vi "Experiment.vi"() -> ()   [LabVIEW 2016]
uses:
  controls/Enum.ctl
  <vilib>/rvi/interface/nirviOpenFPGA/nirviOpenFPGA.xnode
  controls/FPGAVIreferenceTypeDef.ctl
  Course Project/support/Message Queue/Message Queue.lvlib
  <vilib>/rvi/interface/nirviReadWriteControl/nirviReadWriteControl.xnode
  controls/FPGAVIreferenceTypeDefScanEngine.ctl
  <vilib>/FPGAPlugInAG/USB-7856R OEM/niLvFpga_Open_USB-7856R OEM.vi
  FPGA Bitfiles/qnmController797_usbRIO_controllerFPGAmu.lvbitx
  FPGA Bitfiles/lbniAFMControlle_scanControl2_controllerFPGAPX_D62jLejMcas.lvbitx
  controllerFPGA_multiTarget.vi
  <vilib>/FPGAPlugInAG/PXI-7842R/niLvFpga_Open_PXI-7842R.vi
  NiFpgaLv.dll
  <vilib>/rvi/errors/niLvFpgaAdjustHostInterfaceError.vi
  controls/Monitor.ctl
panel:
  in  "Head":i32(listbox)
  in  "Actions":T1
  out "Image":T2
  out "Profileh":dbl[][](graph)
  in  "Scan Engine":i32[](listbox)
  in  "FPGA":i32[](listbox)
  in  "Experiment":i32(listbox)
  in  "Microscope":i32(listbox)
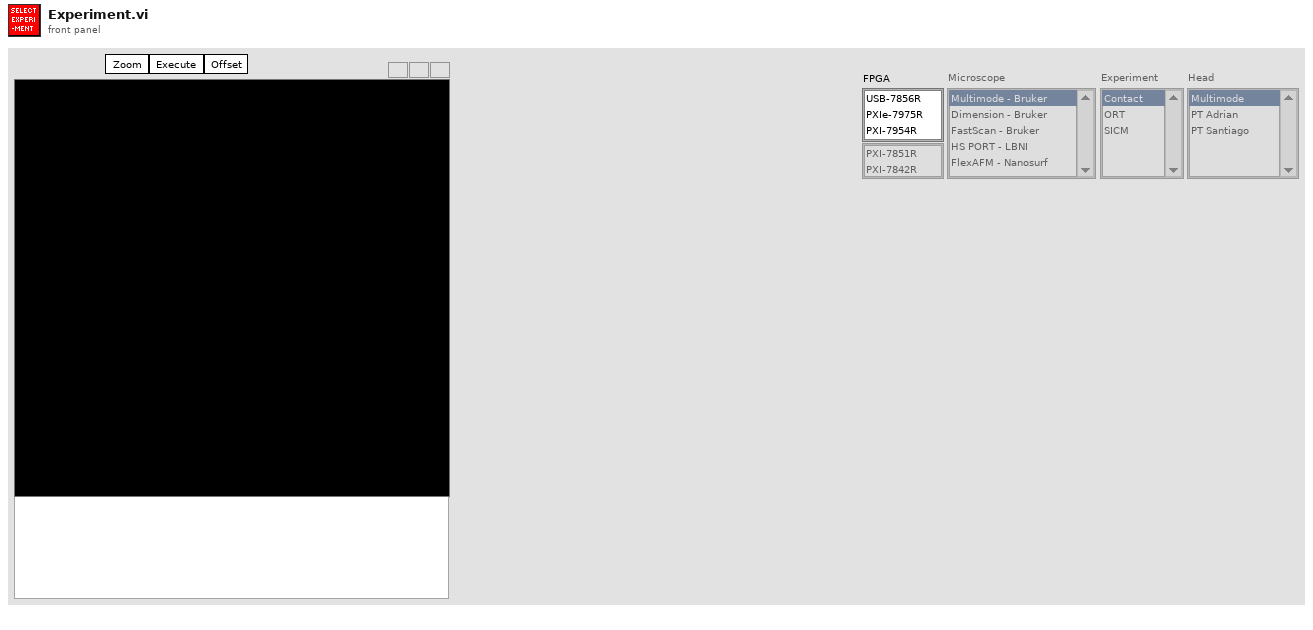
[diagram p1: front panel]
types:
  T1 = cluster{"Zoom":bool, "Execute":bool, "Offset":bool}
  T2 = typedef "Monitor.ctl" = dbl[][]
  T3 = typedef "Message Queue.lvlib/All Message Queues.ctl" = cluster{"IU":refnum<queue>}
  T4 = enum8{"Enabled", "Disabled", "Disabled and Grayed Out"}
  T5 = typedef "Enum.ctl" = enum16{"Init", "Read", "Write"}
  T6 = typedef "FPGAVIreferenceTypeDef.ctl" = refnum<k20>
  T7 = typedef "FPGAVIreferenceTypeDefScanEngine.ctl" = refnum<k20>
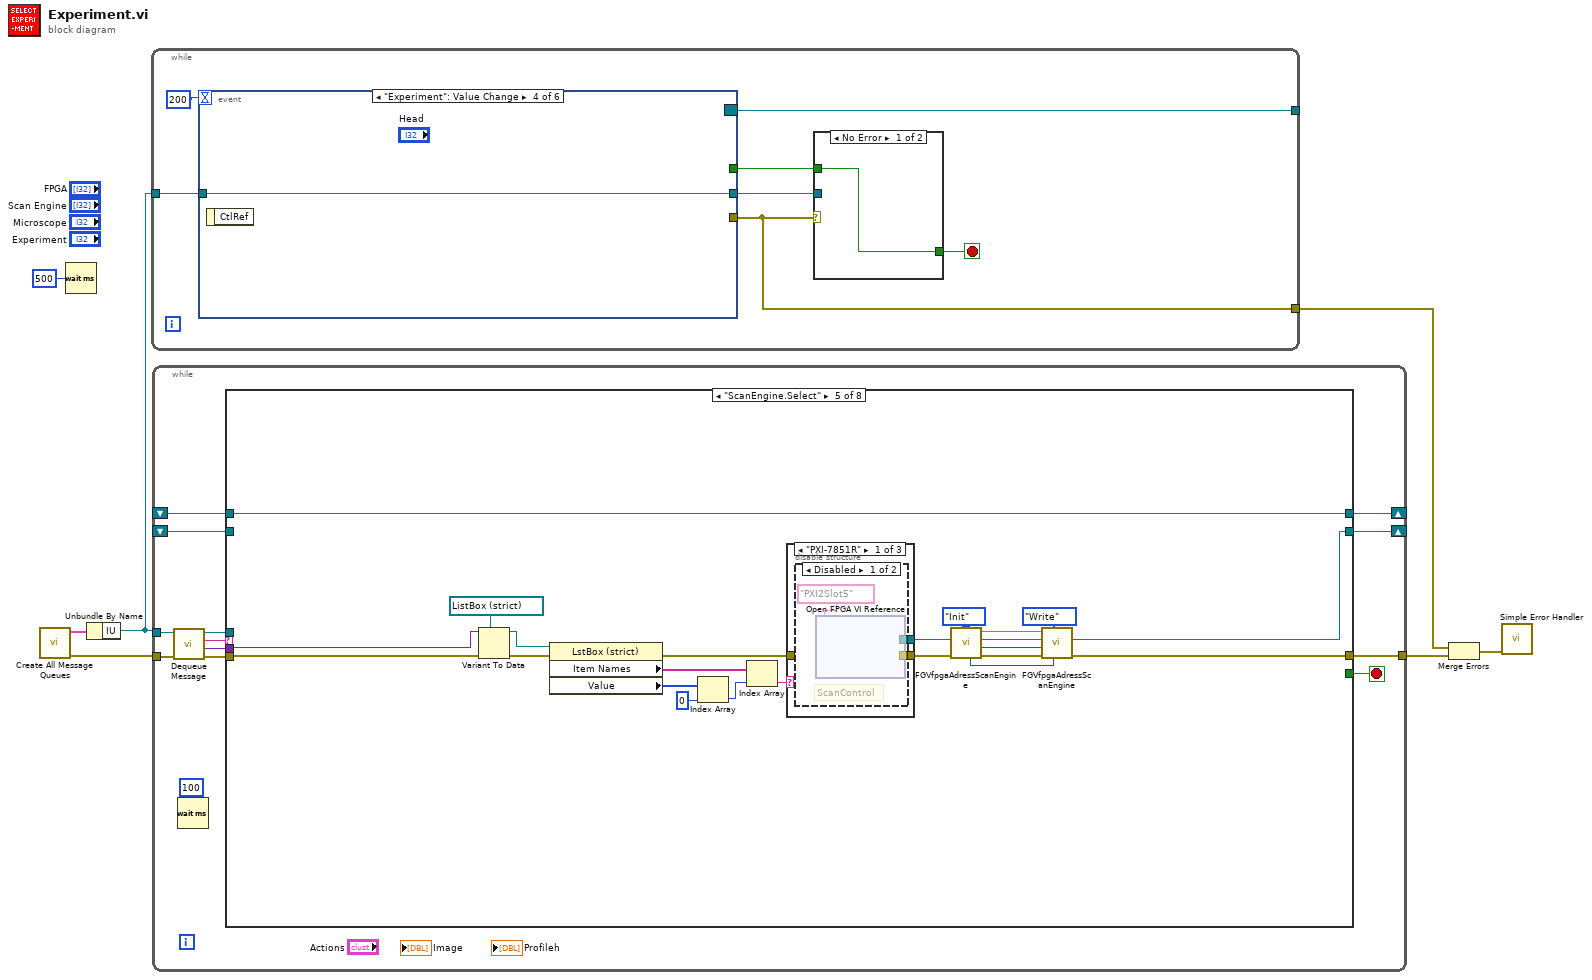
[diagram p0: block diagram]
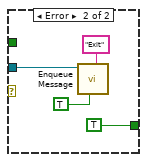
[diagram p2: hidden frame]
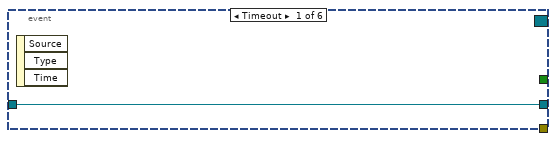
[diagram p3: hidden frame]
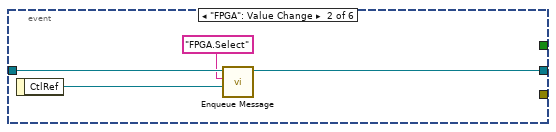
[diagram p4: hidden frame]
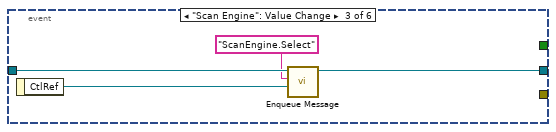
[diagram p5: hidden frame]
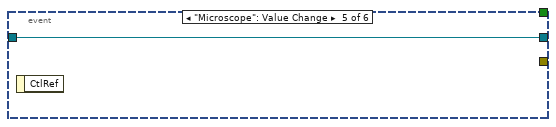
[diagram p6: hidden frame]
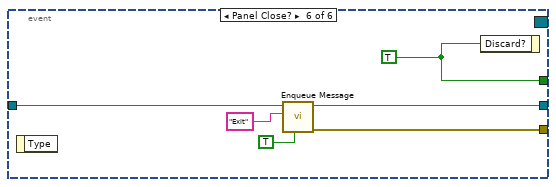
[diagram p7: hidden frame]
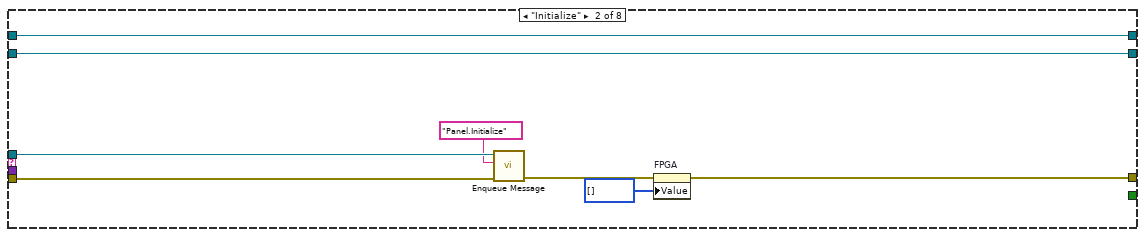
[diagram p9: hidden frame]
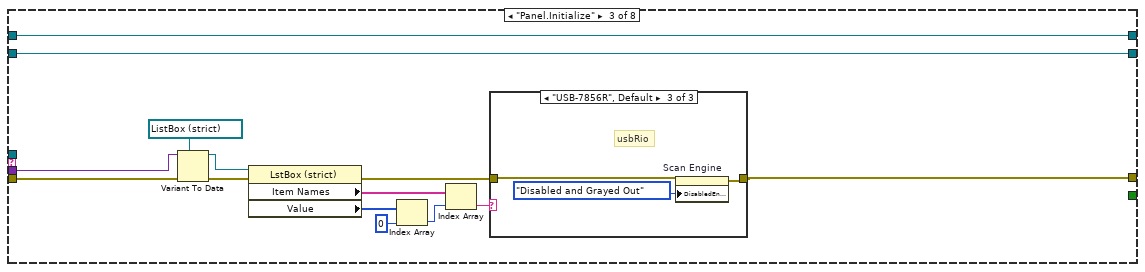
[diagram p10: hidden frame]
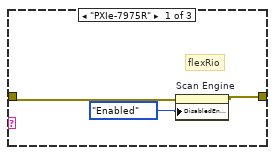
[diagram p11: hidden frame]
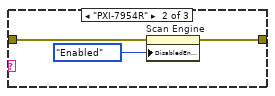
[diagram p12: hidden frame]
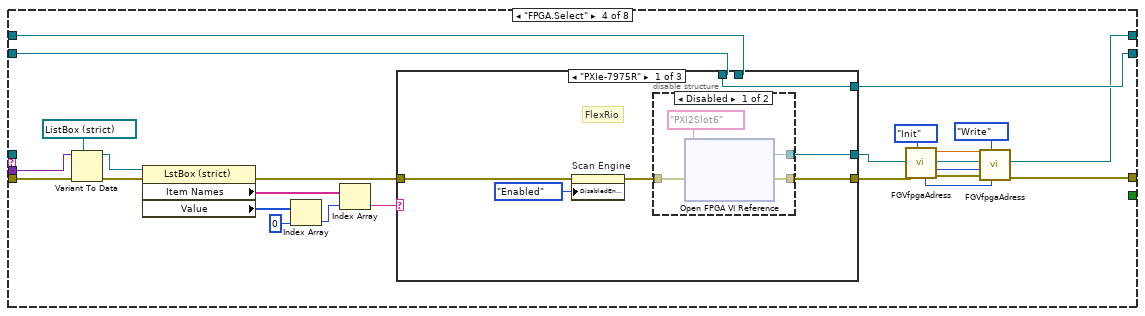
[diagram p13: hidden frame]
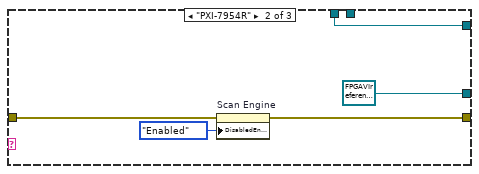
[diagram p15: hidden frame]
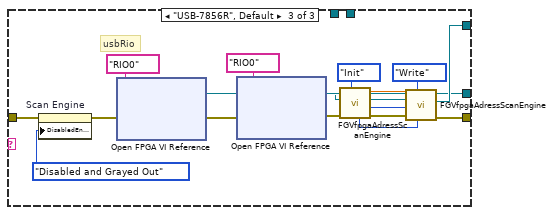
[diagram p16: hidden frame]
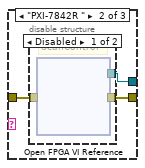
[diagram p18: hidden frame]
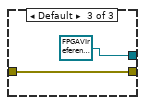
[diagram p20: hidden frame]
diagram:
  n1 = call "Create All Message Queues.vi"() -> ("ErrorOut"=w5:errorcluster, "MessageQueueOut"=w7:T3)  [unwired: 10 in]
  n2 = Wait (ms)(milliseconds to wait=u32 500) -> ()  [unwired: 1 out]
  n3 = Unbundle By Name(w7) -> ("IU"=w6:refnum<queue>)
  n4 = while {
    tunnel: w6 -> [w14]
    tunnel: [w10] -> w1
    tunnel: [w9] -> _
    stop <- w12 stop-if-true
    n5 = event shown="[3] \"Experiment\": Value Change" {
      selector: _ -> [_ _ _ _ _ _]
      dyn-events: [_ _ _ _ _ _] -> w9
      timeout: 200 -> [_ _ _ _ _ _]
      tunnel: [_ _ _ _ _ w36] -> w13
      tunnel: w14 -> [w20 w24 w27 w29 w30 w35]
      tunnel: [_ _ _ _ _ w34] -> w10
      tunnel: [w20 w23 w28 w29 w30 w33] -> w11
      event Timeout {
        n6 = event-data() -> ()  [unwired: 1 in, 3 out]
      }
      event "FPGA": Value Change {
        n7 = event-data() -> ("CtlRef"=w22:refnum<vi>)  [unwired: 1 in]
        n8 = call "Enqueue Message.vi"("Data"=w22, "Message"="FPGA.Select", "Queue"=w24) -> ("Queue dup."=w23:refnum<queue>)  [unwired: 7 in, 1 out]
      }
      event "Scan Engine": Value Change {
        n9 = event-data() -> ("CtlRef"=w25:refnum<vi>)  [unwired: 1 in]
        n10 = call "Enqueue Message.vi"("Data"=w25, "Message"="ScanEngine.Select", "Queue"=w27) -> ("Queue dup."=w28:refnum<queue>)  [unwired: 7 in, 1 out]
      }
      event "Experiment": Value Change {
        n11 = event-data() -> ()  [unwired: 1 in, 1 out]
      }
      event "Microscope": Value Change {
        n12 = event-data() -> ()  [unwired: 1 in, 1 out]
      }
      event Panel Close? {
        w36 = TRUE ("Rejeter ?")
        n13 = event-data() -> ()  [unwired: 1 in, 1 out]
        n14 = call "Enqueue Message.vi"("Prioritary message"=TRUE ("Message prioritaire ? (F)"), "Message"="Exit", "Queue"=w35) -> ("error out"=w34:errorcluster, "Queue dup."=w33:refnum<queue>)  [unwired: 7 in]
        n15 = event-data ("Event Filter Node")("Discard?"=w36) -> ()  [unwired: 1 in, 1 out]
      }
    }
    n16 = case shown="No Error" w10 {
      tunnel: [w15 TRUE ("Rejeter ?")] -> w12
      tunnel: w13 -> [w15 _]
      tunnel: w11 -> [_ w18]
      frame No Error {
      }
      frame Error {
        n17 = call "Enqueue Message.vi"("Prioritary message"=TRUE ("Message prioritaire ? (F)"), "Message"="Exit", "Queue"=w18) -> ()  [unwired: 7 in, 2 out]
      }
    }
  }
  n18 = while {
    tunnel: w6 -> [w43]
    tunnel: w5 -> [w47]
    tunnel: [w48] -> w2
    shift-right: [w40] -> _
    shift-left: _ -> [w39]
    shift-right: [w38] -> _
    shift-left: _ -> [w37]
    stop <- w49 stop-if-true
    n19 = call "Dequeue Message.vi"("entrée d'erreur (pas d'erreur)"=w47, "File d'attente de messages"=w43) -> ("sortie d'erreur"=w46:errorcluster, "Données de message"=w45:variant, "Message"=w42:string, "File d'attente de message dup."=w44:refnum<queue>)  [unwired: 6 in]
    n20 = Wait (ms)(milliseconds to wait=u32 100) -> ()  [unwired: 1 out]
    n21 = case "Conditions des messages" shown="\"ScanEngine.Select\"" w42 {
      selector: w42 -> [_ _ _ _ _ _ _ w206]
      tunnel: w44 -> [_ w60 _ _ _ _ w200 _]
      tunnel: w46 -> [w52 w58 w67 w102 w153 w182 w198 _]
      tunnel: [w52 w54 w64 w93 w154 w190 w197 w204] -> w48
      tunnel: [_ _ _ _ _ _ TRUE _] -> w49
      tunnel: w45 -> [_ _ w63 w101 w152 w181 _ _]
      tunnel: [w51 w57 w62 w91 w148 w188 w196 w202] -> w40
      tunnel: w39 -> [w51 w57 w62 w94 w148 w189 w196 w202]
      tunnel: [w50 w56 w61 w96 w149 w191 w195 w201] -> w38
      tunnel: w37 -> [w50 w56 w61 w95 _ w191 w195 w201]
      frame "--------- Initialization ---------" {
      }
      frame "Initialize" {
        n22 = call "Enqueue Message.vi"("error in"=w58, "Message"="Panel.Initialize", "Queue"=w60) -> ("error out"=w55:errorcluster)  [unwired: 7 in, 1 out]
        n23 = property on="FPGA" class="LstBox (strict)"(error in=w55, "Value"=i32[] [] ("FPGA")) -> (error out=w54:errorcluster)  [unwired: 1 in, 1 out]
      }
      frame "Panel.Initialize" {
        n24 = Variant To Data(error in=w67, type=refnum<vi> refnum ("CtlRef"), Variant=w63) -> (data=w68:refnum<vi>, error out=w69:errorcluster)
        n25 = property class="LstBox (strict)"(reference=w68, error in=w69) -> (error out=w66:errorcluster, "Item Names"=w74:string[], "Value"=w73:i32[])  [unwired: 1 out]
        n26 = Index Array(array=w73, index=0) -> (element=w71:i32)
        n27 = Index Array(array=w74, index=w71) -> (element=w65:string)
        n28 = case shown="\"USB-7856R\", Default" w65 {
          tunnel: [w76 w79 w81] -> w64
          tunnel: w66 -> [w75 w78 w82]
          frame "PXIe-7975R" {
            # "flexRio"
            n29 = property on="Scan Engine" class="LstBox (strict)"(error in=w75, "DisabledEnum"=T4."Enabled" ("Disabled")) -> (error out=w76:errorcluster)  [unwired: 1 in, 1 out]
          }
          frame "PXI-7954R" {
            n30 = property on="Scan Engine" class="LstBox (strict)"(error in=w78, "DisabledEnum"=T4."Enabled" ("Disabled")) -> (error out=w79:errorcluster)  [unwired: 1 in, 1 out]
          }
          frame "USB-7856R", Default {
            # "usbRio"
            n31 = property on="Scan Engine" class="LstBox (strict)"(error in=w82, "DisabledEnum"=T4."Disabled and Grayed Out" ("Disabled")) -> (error out=w81:errorcluster)  [unwired: 1 in, 1 out]
          }
        }
      }
      frame "FPGA.Select" {
        n32 = Variant To Data(error in=w102, type=refnum<vi> refnum ("CtlRef"), Variant=w101) -> (data=w97:refnum<vi>, error out=w99:errorcluster)
        n33 = property class="LstBox (strict)"(reference=w97, error in=w99) -> (error out=w98:errorcluster, "Item Names"=w107:string[], "Value"=w105:i32[])  [unwired: 1 out]
        n34 = Index Array(array=w105, index=0) -> (element=w103:i32)
        n35 = Index Array(array=w107, index=w103) -> (element=w106:string)
        n36 = case shown="\"PXIe-7975R\"" w106 {
          tunnel: [w113 T6 refnum ("FPGA VI Reference Out") w127] -> w92
          tunnel: [w112 w120 w136] -> w89
          tunnel: w98 -> [w110 w119 w139]
          tunnel: [w108 w118 w137] -> w96
          tunnel: w95 -> [w108 w118 _]
          tunnel: w94 -> [_ _ _]
          frame "PXIe-7975R" {
            # "FlexRio"
            n37 = property on="Scan Engine" class="LstBox (strict)"(error in=w110, "DisabledEnum"=T4."Enabled" ("Disabled")) -> (error out=w109:errorcluster)  [unwired: 1 in, 1 out]
            n38 = disable-structure shown="Disabled" {
              disable-tunnel: [w117 _] -> w113
              disable-tunnel: [w116 _] -> w112
              disable-tunnel: w109 -> [w115 _]
              frame Disabled {
                n39 = xnode "Open FPGA VI Reference"("error in"=w115, "resource name"=tag "PXI2Slot6") -> ("FPGA VI Reference Out"=w117:T6, "error out"=w116:errorcluster)
              }
              frame Enabled {
              }
            }
          }
          frame "PXI-7954R" {
            n40 = property on="Scan Engine" class="LstBox (strict)"(error in=w119, "DisabledEnum"=T4."Enabled" ("Disabled")) -> (error out=w120:errorcluster)  [unwired: 1 in, 1 out]
          }
          frame "USB-7856R", Default {
            # "usbRio"
            n41 = property on="Scan Engine" class="LstBox (strict)"(error in=w139, "DisabledEnum"=T4."Disabled and Grayed Out" ("Disabled")) -> (error out=w140:errorcluster)  [unwired: 1 in, 1 out]
            n42 = xnode "Open FPGA VI Reference"("error in"=w140, "resource name"=tag "RIO0") -> ("FPGA VI Reference Out"=w127:T6, "error out"=w125:errorcluster)
            n43 = xnode "Open FPGA VI Reference"("error in"=w125, "resource name"=tag "RIO0") -> ("FPGA VI Reference Out"=w124:T7, "error out"=w123:errorcluster)
            n44 = call "FGVfpgaAdressScanEngine.vi"("Enum"=Enum."Init", "error in"=w123, "FPGA.SEin"=w124) -> ("error out"=w133:errorcluster, "ioFreqHzOut"=w130:u32, "FPGA.SEout"=w128:T7, "voltageRange(+/-)Out"=w131:dbl, "zDataRateOut"=w129:u32)  [unwired: 4 in]
            n45 = call "FGVfpgaAdressScanEngine.vi"("zDataRateIn"=w129, "Enum"=Enum."Write", "error in"=w133, "ioFreqHzIn"=w130, "FPGA.SEin"=w128, "voltageRange(+/-)In"=w131) -> ("error out"=w136:errorcluster, "FPGA.SEout"=w137:T7)  [unwired: 1 in, 3 out]
          }
        }
        n46 = call "FGVfpgaAdress.vi"("Enum"=Enum."Init", "error in"=w89) -> ("error out"=w88:errorcluster, "baseClockOut"=w85:u32, "voltageRange(+/-)Out"=w86:dbl, "ioFreqHzOut"=w84:u32)  [unwired: 4 in, 2 out]
        n47 = call "FGVfpgaAdress.vi"("ioFreqHzIn"=w84, "Enum"=Enum."Write", "error in"=w88, "BaseClockIn"=w85, "FPGA VI Reference In"=w92, "voltageRange(+/-)In"=w86) -> ("error out"=w93:errorcluster, "FPGA VI Reference Out"=w91:T6)  [unwired: 4 out]
      }
      frame "ScanEngine.Select" {
        n48 = Variant To Data(error in=w153, type=refnum<vi> refnum ("CtlRef"), Variant=w152) -> (data=w155:refnum<vi>, error out=w156:errorcluster)
        n49 = property class="LstBox (strict)"(reference=w155, error in=w156) -> (error out=w150:errorcluster, "Item Names"=w162:string[], "Value"=w161:i32[])  [unwired: 1 out]
        n50 = Index Array(array=w161, index=0) -> (element=w159:i32)
        n51 = Index Array(array=w162, index=w159) -> (element=w151:string)
        n52 = case shown="\"PXI-7851R\"" w151 {
          tunnel: [w164 w170 w175] -> w145
          tunnel: w150 -> [_ w169 w175]
          tunnel: [w163 w168 T7 refnum ("FPGAInterfaceIn")] -> w147
          frame "PXI-7851R" {
            n53 = disable-structure shown="Disabled" {
              disable-tunnel: [w167 _] -> w164
              disable-tunnel: [w166 _] -> w163
              frame Disabled {
                # "ScanControl"
                n54 = xnode "Open FPGA VI Reference"("resource name"=tag "PXI2Slot5") -> ("FPGA VI Reference Out"=w166:T7, "error out"=w167:errorcluster)  [unwired: 1 in]
              }
              frame Enabled {
              }
            }
          }
          frame "PXI-7842R " {
            n55 = disable-structure shown="Disabled" {
              disable-tunnel: [w173 _] -> w170
              disable-tunnel: w169 -> [w172 _]
              disable-tunnel: [w171 _] -> w168
              frame Disabled {
                # "ScanControl"
                n56 = xnode "Open FPGA VI Reference"("error in"=w172) -> ("FPGA VI Reference Out"=w171:T7, "error out"=w173:errorcluster)  [unwired: 1 in]
              }
              frame Enabled {
              }
            }
          }
          frame Default {
          }
        }
        n57 = call "FGVfpgaAdressScanEngine.vi"("Enum"=Enum."Init", "error in"=w145) -> ("error out"=w144:errorcluster, "ioFreqHzOut"=w143:u32, "voltageRange(+/-)Out"=w142:dbl, "zDataRateOut"=w141:u32)  [unwired: 5 in, 1 out]
        n58 = call "FGVfpgaAdressScanEngine.vi"("zDataRateIn"=w141, "Enum"=Enum."Write", "error in"=w144, "ioFreqHzIn"=w143, "FPGA.SEin"=w147, "voltageRange(+/-)In"=w142) -> ("error out"=w154:errorcluster, "FPGA.SEout"=w149:T7)  [unwired: 1 in, 3 out]
      }
      frame "Experiment.Select" {
        n59 = Variant To Data(error in=w182, type=refnum<vi> refnum ("CtlRef"), Variant=w181) -> (data=w180:refnum<vi>, error out=w183:errorcluster)
        n60 = property class="LstBox (strict)"(reference=w180, error in=w183) -> (error out=w178:errorcluster, "Item Names"=w187:string[], "Value"=w186:i32[])  [unwired: 1 out]
        n61 = Index Array(array=w186, index=0) -> (element=w184:i32)
        n62 = Index Array(array=w187, index=w184) -> (element=w177:string)
        n63 = case shown="\"Off-Resonance Tapping\"" w177 {
          tunnel: [w192 w193 w194] -> w176
          frame "Off-Resonance Tapping" {
            w192 = u8 1 items=["Contact Mode", "ORT", "Aux"] ("fb.i.source")
          }
          frame "SICM", Default {
            w193 = u8 2 items=["Contact Mode", "ORT", "Aux"] ("fb.i.source")
          }
          frame "Contact" {
            w194 = u8 0 items=["Contact Mode", "ORT", "Aux"] ("fb.i.source")
          }
        }
        n64 = xnode "Read/Write Control"("FPGA VI Reference In"=w189, "error in"=w178, "fb.i.source"=w176) -> ("FPGA VI Reference Out"=w188:T6, "error out"=w190:errorcluster)
      }
      frame "Exit" {
        n65 = Release Queue(queue=w200, error in (no error)=w198) -> (error out=w197:errorcluster)  [unwired: 1 in, 2 out]
      }
      frame Default {
        n66 = Format Into String(format string="The message\"%s\" received in the gestion loop is not valid" ("Texte de message d'erreur inconnu"), w206) -> (resulting string=w203:string)  [unwired: 2 in, 1 out]
        n67 = call <vilib>:"Error Cluster From Error Code.vi"("error message (\"\")"=w203, "error code (0)"=1 ("code d'erreur (0)")) -> ("error out"=w204:errorcluster)  [unwired: 7 in]
      }
    }
  }
  n68 = Merge Errors(w1, w2) -> (w3:errorcluster)
  n69 = call <vilib>:"Simple Error Handler.vi"("error in (no error)"=w3) -> ()  [unwired: 4 in, 5 out]
